vi "encoderOdometry.vi"(6 "Stop.":bool, 9 "angle initial":dbl, 10 "y initial":dbl=250.0, 11 "x initial":dbl=750.0) -> (0 "movement":cluster{dbl[], dbl[]}, 1 "fThetaOdom":dbl=0.5861789702756867, 2 "yfPosOdom":dbl=177.27587822412445, 3 "xfPosOdom":dbl=728.0021187687184)   [LabVIEW 2016]
uses:
  <vilib>/myRIO/Common/Instrument Driver Framework/myRIO v1.0/Encoder/typedefs/Encoder Signal Mode.ctl
  <vilib>/myRIO/Common/Instrument Driver Framework/myRIO v1.0/Encoder/typedefs/Encoder Channels Enum.ctl
  <vilib>/myRIO/Common/Instrument Driver Framework/Utilities/typedefs/Generic FPGA Reference.ctl
  <vilib>/myRIO/Common/Instrument Driver Framework/Utilities/typedefs/myRIO v1.0 Reference.ctl
  <vilib>/myRIO/Common/Instrument Driver Framework/Utilities/typedefs/Hardware Version Enum.ctl
  <vilib>/myRIO/Common/Instrument Driver Framework/Utilities/typedefs/myRIO Generic Hardware Reference.ctl
  <vilib>/myRIO/Instrument Drivers/Onboard IO/Encoder/typedefs/Encoder Reference.ctl
  <vilib>/myRIO/Instrument Drivers/Onboard IO/Encoder/Encoder.lvlib
  <vilib>/myRIO/Instrument Drivers/Onboard IO/Encoder/vis/Read.vi
  <vilib>/myRIO/Common/Instrument Driver Framework/myRIO v1.0/Encoder/typedefs/Encoder Configuration v1.0.ctl
  <vilib>/userdefined/High Color/nirio_resource_hc.ctl
  <vilib>/myRIO/Common/Instrument Driver Framework/myRIO v1.0/Encoder/vis/myRIO v1.1 Open Encoder.vi
  <vilib>/myRIO/Common/Instrument Driver Framework/myRIO v1.0/Encoder/vis/myRIO v1.0 Configure Encoder.vi
  <vilib>/myRIO/Instrument Drivers/Onboard IO/Encoder/vis/myRIO Encoder Open.xnode
  <vilib>/myRIO/Common/Instrument Driver Framework/Utilities/vis/Is FPGA Ref Available.vi
  <vilib>/myRIO/Express VI/Onboard IO/Encoder/Encoder Express VI.xnode
panel:
  in  "width":dbl=263.0
  in  "wheelDia":dbl=100.0
  # "Latest values for robot location"
  # "Initial values for robot location"
  # "Terminate Loop"
  # "Initial x value in mm"
  # "Latest x value in mm"
  # "Center to center distance\nof wheels in mm"
  # "Initial y value in mm"
  # "Latest y value in mm"
  # "Wheel diametre in mm"
  # "Initial angle in degrees"
  # "Latest angle in radians"
  # "Cluster of arrays depicting the path of the robot"
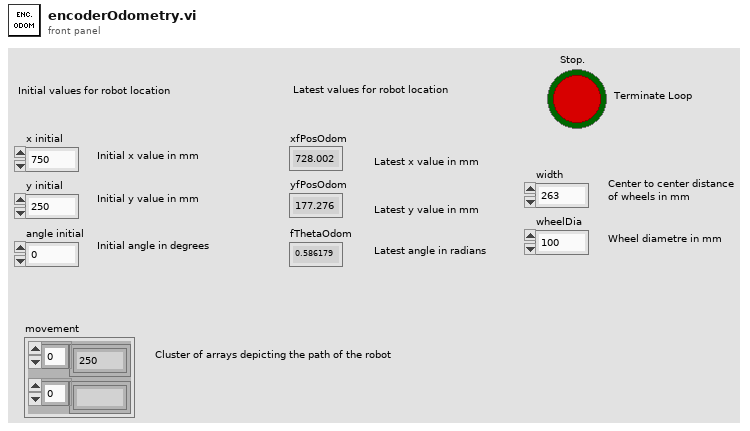
[diagram p1: front panel]
types:
  T1 = typedef "Encoder.lvlib/Encoder Reference.ctl" = cluster{"myRIO Reference":T2, "Encoder Channels Enum":T6}
  T2 = typedef "myRIO Generic Hardware Reference.ctl" = cluster{"myRIO Model":T3, "myRIO Hardware Reference":T4}
  T3 = typedef "Hardware Version Enum.ctl" = enum16{"Unknown", "myRIO-1900", "myRIO-1950", "roboRIO", "NI ELVIS RIO CM"}
  T4 = typedef "myRIO v1.0 Reference.ctl" = cluster{"Generic FPGA Reference":T5, "Allow multiple opens":bool}
  T5 = typedef "Generic FPGA Reference.ctl" = refnum<k20>
  T6 = typedef "Encoder Channels Enum.ctl" = enum16{"Not Connected", "C/ENC0", "C/ENC1", "A/ENC", "B/ENC", "DIO/ENC0", "DIO/ENC1", "DIO/ENC2", "DIO/ENC3", "DIO/ENC4"}
  T7 = typedef "Encoder Signal Mode.ctl" = enum16{"Quadrature phase signal", "Step and direction signal"}
  T8 = typedef "nirio_resource_hc.ctl" = tag
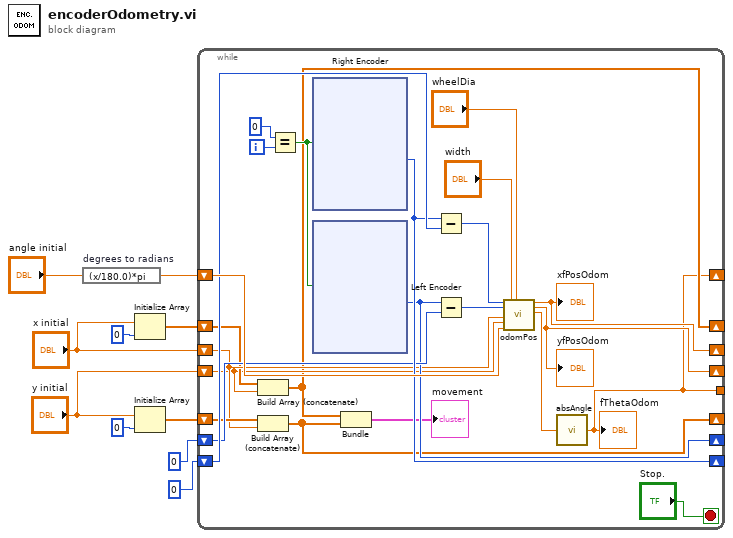
[diagram p0: block diagram]
diagram:
  n1 = expression code="(x/180.0)*pi" "degrees to radians"("angle initial") -> (w3:dbl)
  n2 = Initialize Array("x initial", 0 ("dimension size")) -> (w10:dbl[])
  n3 = Initialize Array("y initial", 0 ("dimension size")) -> (w8:dbl[])
  n4 = while {
    shift-right: [w12] -> _
    shift-left: "y initial" -> [w19]
    shift-right: [w13] -> _
    shift-left: "x initial" -> [w21]
    shift-right: [w11] -> _
    shift-left: w3 -> [w31]
    shift-right: [w25] -> _
    shift-left: 0 ("Counter Value") -> [w26]
    shift-right: [w28] -> _
    shift-left: 0 ("Counter Value") -> [w30]
    shift-right: [w15] -> _
    shift-left: w10 -> [w20]
    shift-right: [w16] -> _
    shift-left: w8 -> [w22]
    tunnel: [w11] -> _
    i -> [w34]
    stop <- "Stop." stop-if-true
    n5 = Build Array (concatenate)(w20, w19) -> (w15:dbl[])
    n6 = Build Array (concatenate)(w22, w21) -> (w16:dbl[])
    n7 = Equal?(x=0, y=w34) -> (x = y?=w32:bool)
    n8 = xnode "Right Encoder"("Reset Counter"=w32) -> ("Counter Value"=w28:i32)  [unwired: 1 in, 3 out]
    n9 = xnode "Left Encoder"("Reset Counter"=w32) -> ("Counter Value"=w25:i32)  [unwired: 1 in, 3 out]
    n10 = Bundle(w15, w16) -> (→"movement":cluster{dbl[], dbl[]})  [unwired: 1 in]
    n11 = Subtract(x=w28, y=w30) -> (x-y=w29:i32)
    n12 = Subtract(x=w25, y=w26) -> (x-y=w27:i32)
    n13 = call "odomPos.vi"("dLeft"=w29, "dRight"=w27, "xiPos"=w21, "yiPos"=w19, "iTheta"=w31, "width"="width", "wheelDia"="wheelDia") -> ("xfPos"=w13:dbl, "yfPos"=w12:dbl, "fTheta"=w18:dbl)  [unwired: 10 in]
    "xfPosOdom" <- w13
    "yfPosOdom" <- w12
    n14 = call "absAngle.vi"("Numeric"=w18) -> ("Numeric 2"=w11:dbl)  [unwired: 4 in]
    "fThetaOdom" <- w11
  }
